vi "Auto Check Winch.vi"(11 "Run?":bool) -> (3 "Done":bool)   [LabVIEW 2013]
uses:
  Globals/Homes.vi
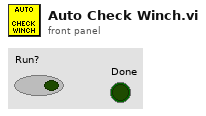
[diagram p1: front panel]
types:
  T1 = typedef "WPI_AnalogChannelDevRef.ctl" = cluster{"DevStatus":errorcluster, "Analog Module":T2, "Analog Channel":T3}
  T2 = typedef "FPGA_TypedefAnalogModule.ctl" = enum16{"Analog Module 1", "Analog Module 2"}
  T3 = typedef "FPGA_AIChannel.ctl" = enum8{"AI 1", "AI 2", "AI 3", "AI 4", "AI 5", "AI 6", "AI 7", "AI 8", "Invalid"}
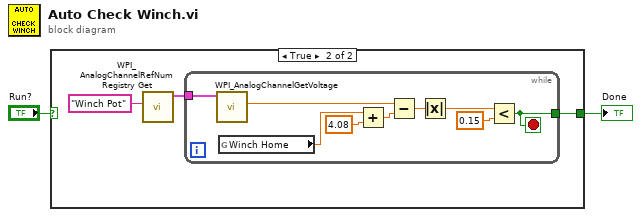
[diagram p0: block diagram]
diagram:
  n1 = case shown="True" "Run?" {
    selector: "Run?" -> [w3 _]
    tunnel: [w3 w4] -> w1
    frame False {
    }
    frame True {
      n2 = call <vilib>:"WPI_AnalogChannelRefNum Registry Get.vi"("refnum name"="Winch Pot") -> ("AIDeviceRef"=w6:T1)  [unwired: 9 in, 1 out]
      n3 = while {
        tunnel: w6 -> [w15]
        tunnel: [w7] -> w4
        stop <- w7 stop-if-true
        n4 = call <vilib>:"WPI_AnalogChannelGetVoltage.vi"("AIDeviceRef"=w15) -> ("Voltage"=w14:dbl)  [unwired: 8 in, 2 out]
        n5 = global read "Homes.vi" "Winch Home"() -> (w11:dbl)
        n6 = Add(x=w11, y=4.08) -> (x+y=w12:dbl)
        n7 = Subtract(x=w14, y=w12) -> (x-y=w13:dbl)
        n8 = Absolute Value(x=w13) -> (abs(x)=w9:dbl)
        n9 = Less?(x=w9, y=0.15) -> (x < y?=w7:bool)
      }
    }
  }
  "Done" <- w1
